vi "Autonomous Independent.vi"   [LabVIEW 2015]
doc: "This VI is called when autonomous begins, and will automatically be terminated when autonomous ends. You can carry out timed or sensor driven robot movement independently without needing to return to the caller."
uses:
  <vilib>/Rock Robotics/WPI/SafetyOutput/WPI_SafetyOutputConfigMenu.ctl
  <vilib>/Rock Robotics/Network Tables/NT Read String.vi
  <vilib>/Rock Robotics/WPI/Utilities/WPI_GetSetVariantRefNum.vi
  <vilib>/addons/control/pid/pid.llb/PID (DBL).vi
  <vilib>/Rock Robotics/WPI/RobotDrive/WPI_RobotDriveArcadeDrive_Standard(NoSaturation).vi
  <vilib>/Rock Robotics/Network Tables/NT Write Numeric Array.vi
  Z navX/navX Library v2/navX Library v2.lvlib
  <vilib>/addons/control/pid/NI_PID_pid.lvlib
panel:
  # "Be sure to right-click and choose Data Operations>>Make Current Value default if you want to save the array values with the VI"
types:
  T1 = cluster{"proportional gain (Kc)":dbl, "integral time (Ti, min)":dbl, "derivative time (Td, min)":dbl}
  T2 = typedef "WPI_SafetyOutputConfigMenu.ctl" = enum16{"Enable", "Disable"}
  T3 = typedef "navX Library v2.lvlib/Z900_navX_DeviceTypeDef.ctl" = cluster{"Interface":cluster{"Protocol":T4, "Update Rate (4Hz-60Hz)":u8, "navX Open TypeDef":variant}, "Notify Packet":refnum<notifier>, "Loop VI Refnum":refnum<vi>, "Ready to Close Occurrence Refnum":refnum<k4>}
  T4 = typedef "navX Library v2.lvlib/Z900_navX_ProtocolTypeDef.ctl" = enum16{"SERIAL", "I2C", "SPI"}
  T5 = cluster{"LinearAcceleration X":dbl, "LinearAcceleration Y":dbl, "LinearAcceleration Z":dbl}
  T6 = cluster{"Velocity X":dbl, "Velocity Y":dbl, "Velocity Z":dbl, "Displacement X":dbl, "Displacement Y":dbl, "Displacement Z":dbl}
  T7 = cluster{"Yaw":dbl, "Roll":dbl, "Pitch":dbl, "Heading":dbl, "Fused Heading":dbl}
  T8 = typedef "WPI_RobotDriveDevRef.ctl" = cluster{"DevStatus":errorcluster, "Motors[]":T9[], "Square Inputs":bool, "Max Output":dbl}
  T9 = typedef "WPI_MotorControlDeviceRef.ctl" = cluster{"DeviceStatus":errorcluster, "Type":T10, "PWM":cluster{"PWM Channel":T11, "DeadBand":T12}, "CAN":cluster{"Device Number":u8, "Control Mode":T13, "Semaphore":T14, "Max Vout":dbl, "TalonSRX Control Mode":T15}, "Invert":bool}
  T10 = typedef "WPI_MotorControlType.ctl" = enum16{"PWM", "CAN", "CANTalonSRX"}
  T11 = typedef "FPGA_DIOPWMChannel.ctl" = enum8{"PWM 0", "PWM 1", "PWM 2", "PWM 3", "PWM 4", "PWM 5", "PWM 6", "PWM 7", "PWM 8", "PWM 9", "PWM MXP 0", "PWM MXP 1", "PWM MXP 2", "PWM MXP 3", "PWM MXP 4", "PWM MXP 5", "PWM MXP 6", "PWM MXP 7", "PWM MXP 8", "PWM MXP 9", "Invalid"}
  T12 = typedef "WPI_PWMDeadband.ctl" = cluster{"Name":string, "maxPositivePwm":i32, "minPositivePwm":i32, "centerPwm":i32, "maxNegativePwm":i32, "minNegativePwm":i32, "angularRange":u16}
  T13 = typedef "WPI_CANJaguar_ControlMode.ctl" = enum8{"Percent VBus", "Current", "Speed", "Position", "Voltage"}
  T14 = typedef "Semaphore RefNum" = refnum<k1>
  T15 = typedef "WPI_CANTalonSRX_APIControlMode.ctl" = enum8{"Percent VBus", "Speed", "Position", "Slave", "Unchanged / Invalid", "Voltage Compensation", "Current", "Motion Profile"}
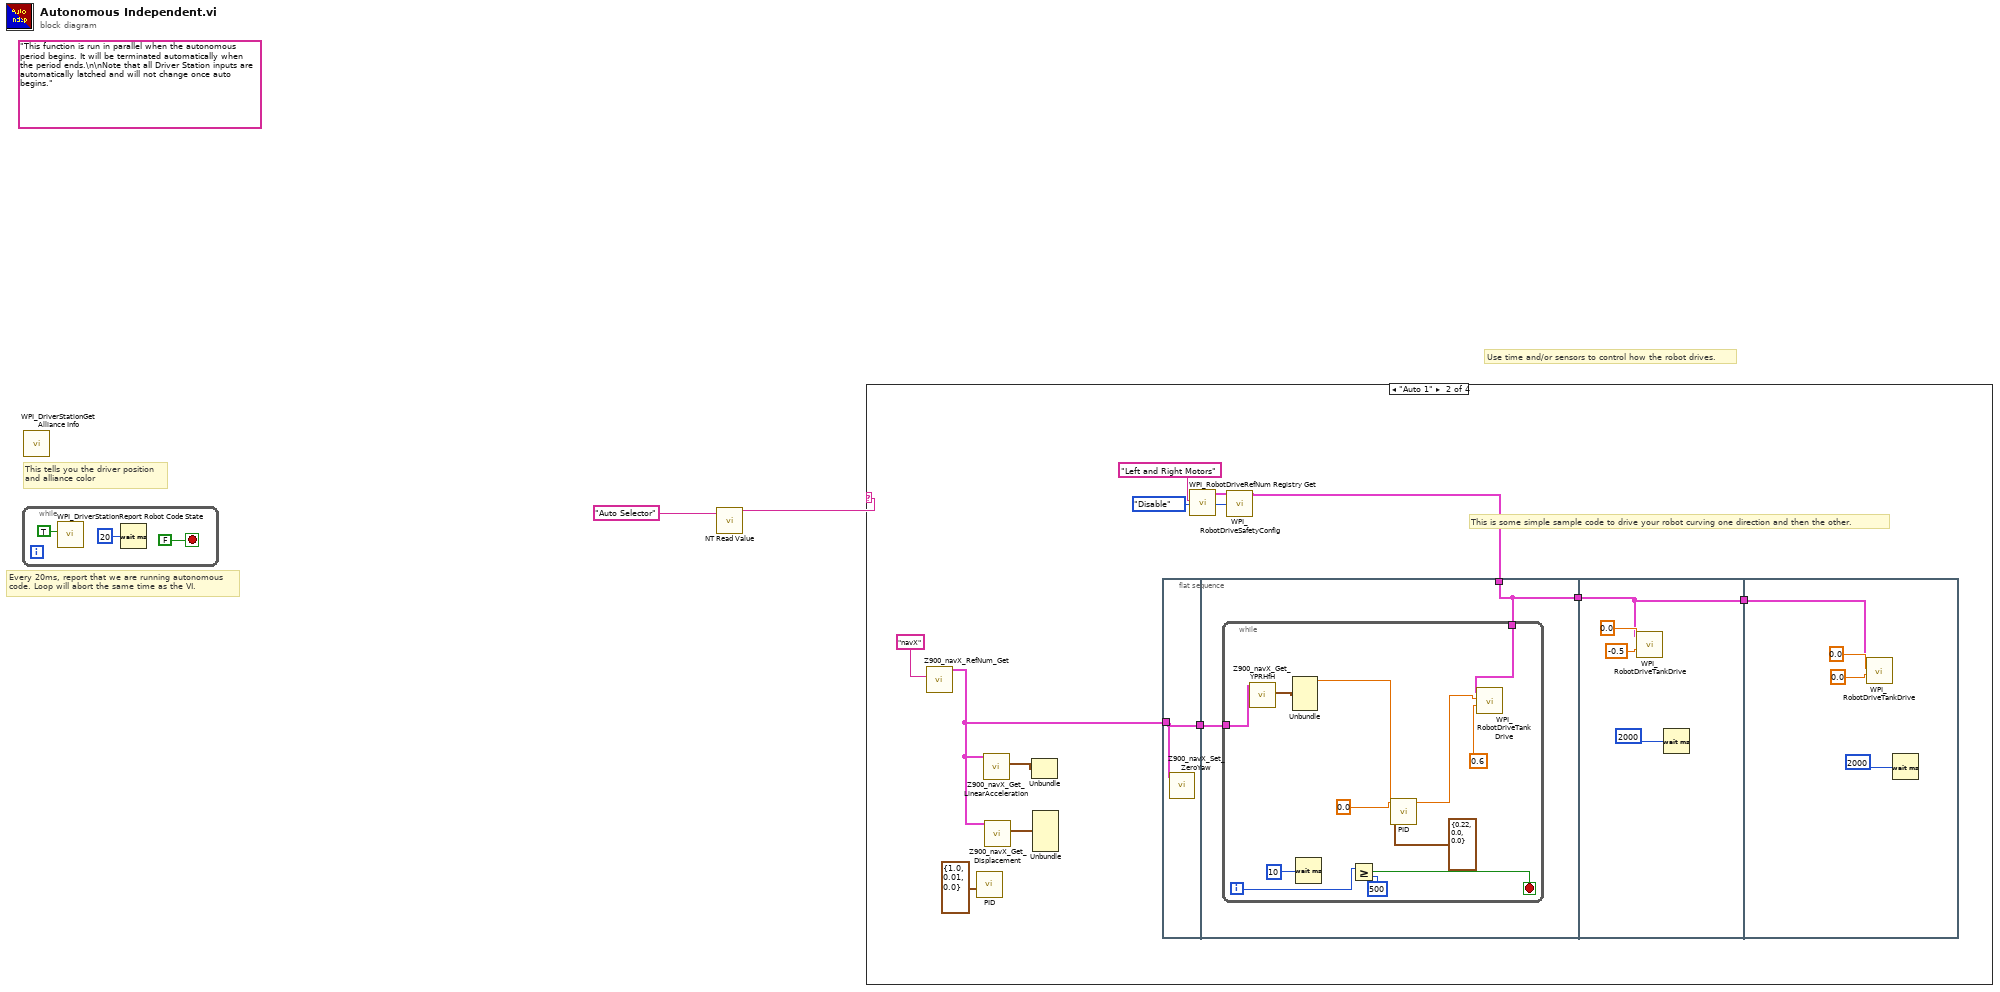
[diagram p0: block diagram]
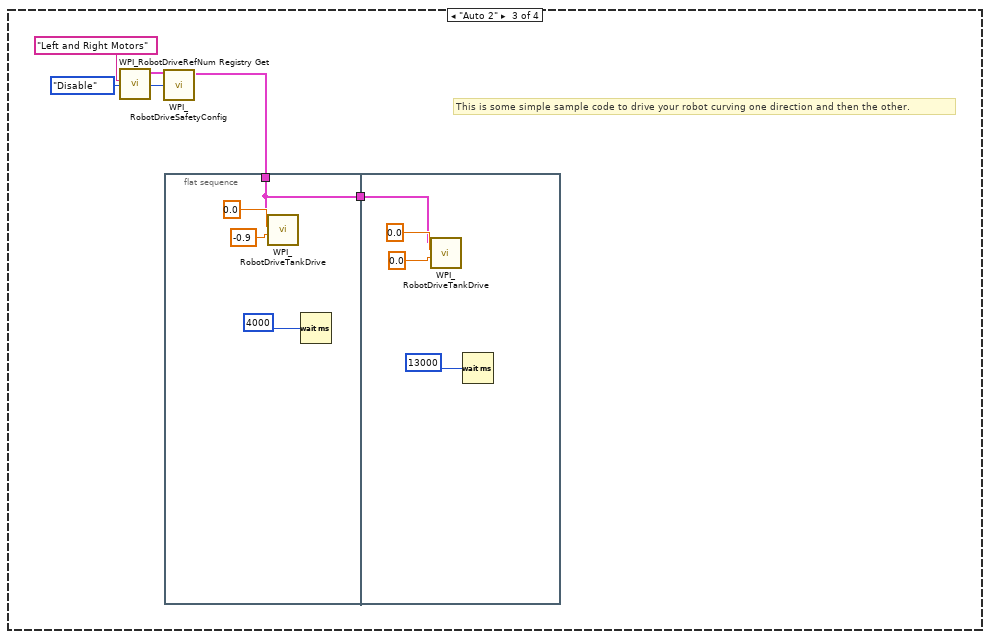
[diagram p3: hidden frame]
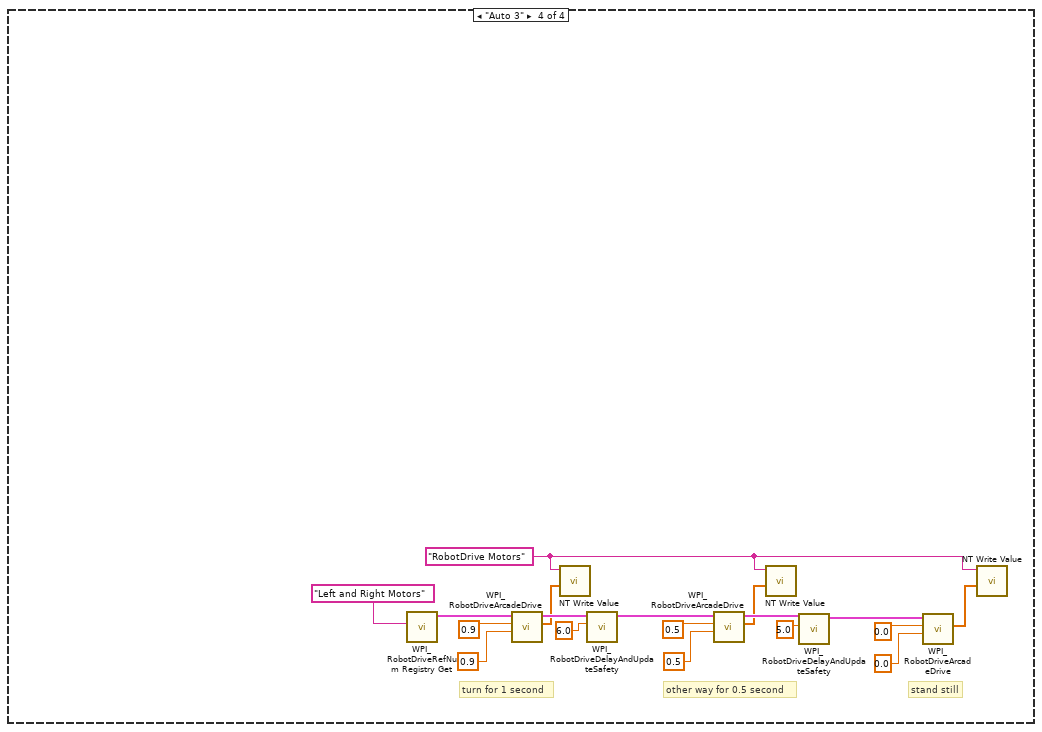
[diagram p4: hidden frame]
diagram:
  (unwired) "This function is run in parallel when the autonomous period begins. It will be terminated automatically when the period ends.\n\nNote that all Driver Station inputs are automatically latched and will not change once auto begins."
  # "Use time and/or sensors to control how the robot drives."
  # "Every 20ms, report that we are running autonomous\ncode. Loop will abort the same time as the VI."
  # "This tells you the driver position\nand alliance color"
  n1 = while {
    stop <- FALSE stop-if-true
    n2 = call <vilib>:"WPI_DriverStationReport Robot Code State.vi"("Autonomous"=TRUE) -> ()  [unwired: 10 in, 1 out]
    n3 = Wait (ms)(milliseconds to wait=u32 20) -> ()  [unwired: 1 out]
  }
  n4 = call <vilib>:"WPI_DriverStationGet Alliance Info.vi"() -> ()  [unwired: 12 out]
  n5 = call-poly <vilib>:"NT Read Value.vi"("Name"="Auto Selector") -> ("String"=w1:string)  [unwired: 9 in, 1 out]
  n6 = case shown="\"Auto 1\"" w1 {
    frame Default {
      # "You can put your main auto here, or you can right-click on the case and make any\nother frame be the default case."
      # "This is the frame that will execute if no selection is made, or if it is not recognized"
    }
    frame "Auto 1" {
      # "This is some simple sample code to drive your robot curving one direction and then the other."
      n7 = call "Z900_navX_RefNum_Get.vi"("refnum name"="navX") -> ("navX Device"=w8:T3)  [unwired: 9 in, 1 out]
      n8 = call-poly <vilib>:"PID.vi"("PID gains"=T1 {"proportional gain (Kc)"=1.0, "integral time (Ti, min)"=0.01, "derivative time (Td, min)"=0.0}) -> ()  [unwired: 9 in, 2 out]
      n9 = call "Z900_navX_Get_LinearAcceleration.vi"("navX Device"=w8) -> ("Linear Acceleration"=w10:T5)  [unwired: 7 in, 3 out]
      n10 = call "Z900_navX_Get_Displacement.vi"("navX Device"=w8) -> ("Displacement"=w9:T6)  [unwired: 7 in, 3 out]
      n11 = Unbundle(w10) -> ()  [unwired: 3 out]
      n12 = Unbundle(w9) -> ()  [unwired: 6 out]
      n13 = flat-sequence {
        tunnel: w8 -> [w18]
        tunnel: [w18] -> w6
        tunnel: w13 -> [w20]
        tunnel: [w20] -> w17
        tunnel: w6 -> [w19]
        tunnel: w17 -> [w33]
        tunnel: [w33] -> w12
        tunnel: w12 -> [w37]
        frame #0 {
          n14 = call "Z900_navX_Set_ZeroYaw.vi"("navX Device"=w18) -> ()  [unwired: 9 in, 2 out]
        }
        frame #1 {
          n15 = while {
            tunnel: w20 -> [w29]
            tunnel: w19 -> [w23]
            i -> [w28]
            stop <- w26 stop-if-true
            n16 = call "Z900_navX_Get_YPRHfH.vi"("navX Device"=w23) -> ("YRPHfH"=w25:T7)  [unwired: 7 in, 3 out]
            n17 = Unbundle(w25) -> ("Yaw"=w24:dbl)  [unwired: 4 out]
            n18 = Wait (ms)(milliseconds to wait=10) -> ()  [unwired: 1 out]
            n19 = Greater Or Equal?(x=w28, y=500) -> (x >= y?=w26:bool)
            n20 = call-poly <vilib>:"PID.vi"("PID gains"=T1 {"proportional gain (Kc)"=0.22, "integral time (Ti, min)"=0.0, "derivative time (Td, min)"=0.0}, "process variable"=w24, "setpoint"=0.0) -> ("output"=w21:dbl)  [unwired: 7 in, 1 out]
            n21 = call <vilib>:"WPI_RobotDriveTankDrive.vi"("Right axis value"=0.6, "Left axis value"=w21, "RobotDriveDevRef"=w29) -> ()  [unwired: 6 in, 3 out]
          }
        }
        frame #2 {
          n22 = call <vilib>:"WPI_RobotDriveTankDrive.vi"("Right axis value"=-0.5, "Left axis value"=0.0, "RobotDriveDevRef"=w33) -> ()  [unwired: 6 in, 3 out]
          n23 = Wait (ms)(milliseconds to wait=2000) -> ()  [unwired: 1 out]
        }
        frame #3 {
          n24 = call <vilib>:"WPI_RobotDriveTankDrive.vi"("Right axis value"=0.0, "Left axis value"=0.0, "RobotDriveDevRef"=w37) -> ()  [unwired: 6 in, 3 out]
          n25 = Wait (ms)(milliseconds to wait=2000) -> ()  [unwired: 1 out]
        }
      }
      n26 = call <vilib>:"WPI_RobotDriveRefNum Registry Get.vi"("refnum name"="Left and Right Motors") -> ("RobotDriveDevRef"=w14:T8)  [unwired: 9 in, 1 out]
      n27 = call <vilib>:"WPI_RobotDriveSafetyConfig.vi"("mode"=WPI_SafetyOutputConfigMenu."Disable", "RobotDriveDevRef"=w14) -> ("RobotDriveDevRef"=w13:T8)  [unwired: 8 in, 1 out]
    }
    frame "Auto 2" {
      # "This is some simple sample code to drive your robot curving one direction and then the other."
      n28 = call <vilib>:"WPI_RobotDriveRefNum Registry Get.vi"("refnum name"="Left and Right Motors") -> ("RobotDriveDevRef"=w43:T8)  [unwired: 9 in, 1 out]
      n29 = call <vilib>:"WPI_RobotDriveSafetyConfig.vi"("mode"=WPI_SafetyOutputConfigMenu."Disable", "RobotDriveDevRef"=w43) -> ("RobotDriveDevRef"=w42:T8)  [unwired: 8 in, 1 out]
      n30 = flat-sequence {
        tunnel: w42 -> [w46]
        tunnel: [w46] -> w41
        tunnel: w41 -> [w51]
        frame #0 {
          n31 = call <vilib>:"WPI_RobotDriveTankDrive.vi"("Right axis value"=-0.9, "Left axis value"=0.0, "RobotDriveDevRef"=w46) -> ()  [unwired: 6 in, 3 out]
          n32 = Wait (ms)(milliseconds to wait=4000) -> ()  [unwired: 1 out]
        }
        frame #1 {
          n33 = call <vilib>:"WPI_RobotDriveTankDrive.vi"("Right axis value"=0.0, "Left axis value"=0.0, "RobotDriveDevRef"=w51) -> ()  [unwired: 6 in, 3 out]
          n34 = Wait (ms)(milliseconds to wait=13000) -> ()  [unwired: 1 out]
        }
      }
    }
    frame "Auto 3" {
      w55 = "RobotDrive Motors" ("Name")
      # "stand still"
      # "other way for 0.5 second"
      # "turn for 1 second"
      n35 = call <vilib>:"WPI_RobotDriveRefNum Registry Get.vi"("refnum name"="Left and Right Motors") -> ("RobotDriveDevRef"=w71:T8)  [unwired: 1 in, 9 out]
      n36 = call-poly <vilib>:"WPI_RobotDriveArcadeDrive.vi"("Y axis value"=0.9 ("X axis value"), "X axis value"=0.9, "RobotDriveDevRef"=w71) -> ("Motor Values"=w54:dbl[], "RobotDriveDevRef"=w64:T8)  [unwired: 1 in, 6 out]
      n37 = call-poly <vilib>:"NT Write Value.vi"("Numeric Array"=w54, "Name"=w55) -> ()  [unwired: 9 in, 1 out]
      n38 = call <vilib>:"WPI_RobotDriveDelayAndUpdateSafety.vi"("Delay (s)"=6.0, "RobotDriveDevRef"=w64) -> ("RobotDriveDevRef 2"=w65:T8)  [unwired: 8 in, 1 out]
      n39 = call-poly <vilib>:"WPI_RobotDriveArcadeDrive.vi"("Y axis value"=0.5 ("X axis value"), "X axis value"=0.5, "RobotDriveDevRef"=w65) -> ("Motor Values"=w56:dbl[], "RobotDriveDevRef"=w66:T8)  [unwired: 1 in, 6 out]
      n40 = call-poly <vilib>:"NT Write Value.vi"("Numeric Array"=w56, "Name"=w55) -> ()  [unwired: 9 in, 1 out]
      n41 = call <vilib>:"WPI_RobotDriveDelayAndUpdateSafety.vi"("Delay (s)"=5.0, "RobotDriveDevRef"=w66) -> ("RobotDriveDevRef 2"=w67:T8)  [unwired: 8 in, 1 out]
      n42 = call-poly <vilib>:"WPI_RobotDriveArcadeDrive.vi"("Y axis value"=0.0 ("X axis value"), "X axis value"=0.0, "RobotDriveDevRef"=w67) -> ("Motor Values"=w57:dbl[])  [unwired: 1 in, 7 out]
      n43 = call-poly <vilib>:"NT Write Value.vi"("Numeric Array"=w57, "Name"=w55) -> ()  [unwired: 9 in, 1 out]
    }
  }
